vi "En.vi"(1 "Turn-table Centre (Xm)":dbl, 2 "Equivalent Nozzle Radius (Rn)":dbl, 3 "Nozzle Blockage Factor (Eq)":dbl) -> (0 "Nozzle Blockage Correction (En)":dbl)   [LabVIEW 2017]
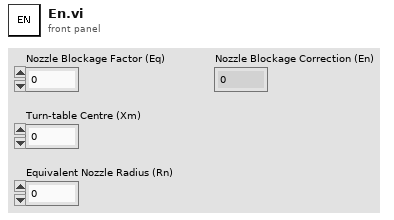
[diagram p1: front panel]
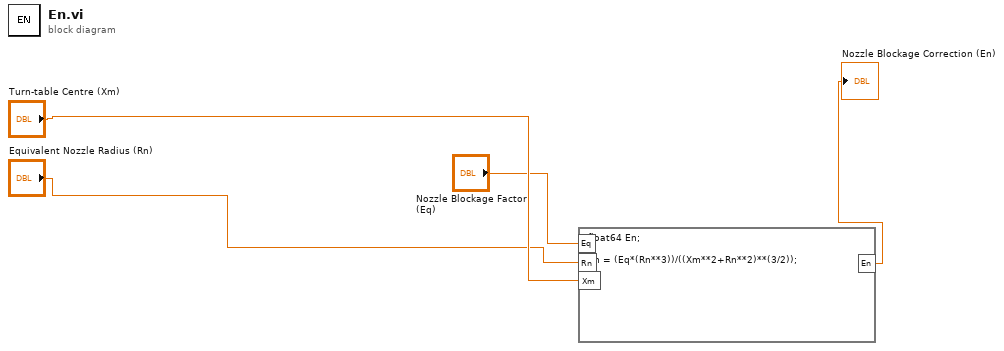
[diagram p0: block diagram]
diagram:
  n1 = formula code="float64 En;\n\nEn = (Eq*(Rn**3))/((Xm**2+Rn**2)**(3/2));"("Eq"="Nozzle Blockage Factor (Eq)", "Rn"="Equivalent Nozzle Radius (Rn)", "Xm"="Turn-table Centre (Xm)") -> ("En"=→"Nozzle Blockage Correction (En)":dbl)
